vi "Set ADC.vi"(8 "error in (no error)":errorcluster, 9 "Data Rate":T1, 10 "Configure NAU7802":T2={"PGA"=enum."x1", "LDOVoltage"=enum."2.7"}, 11 "NAU7802 in":refnum<class "Adafruit NAU7802 24bit Strain Gauge.lvclass">) -> (0 "error out":errorcluster, 3 "NAU7802 out":refnum<class "Adafruit NAU7802 24bit Strain Gauge.lvclass">)   [LabVIEW 2020, in "CTI-Peripheral.lvlib" / "Adafruit NAU7802 24bit Strain Gauge.lvclass"]
uses:
  Adafruit NAU7802 24bit Strain Gauge.lvclass
  Private/ConfigData.ctl
  Private/NAU7802PGA.ctl
  Private/NAU7802LDOVoltage.ctl
  Private/NAU7802DataRate.ctl
  Adafruit NAU7802 24bit Strain Gauge.lvclass/Adafruit NAU7802 24bit Strain Gauge.ctl
  CTI/I2C Connection/I2C Connection.lvclass/I2C Connection.ctl
  CTI/Session/I2C Write Data.vi
  CTI/Session/I2C Read Data.vi
  CTI/I2C Connection/I2C Connection.lvclass
panel:
  out "Data":string
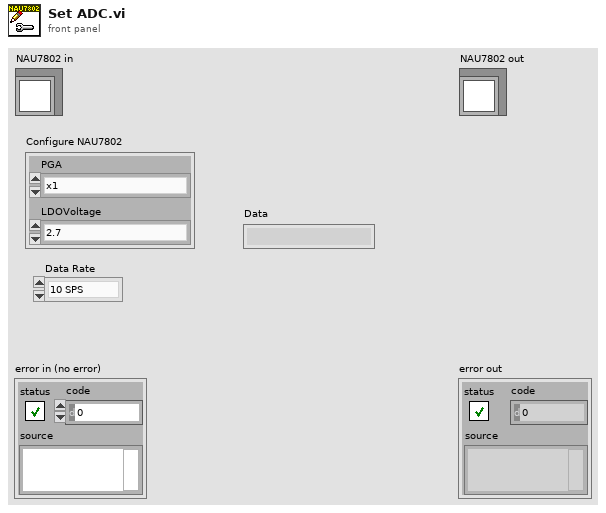
[diagram p1: front panel]
types:
  T1 = typedef "CTI-Peripheral.lvlib/Adafruit NAU7802 24bit Strain Gauge.lvclass/NAU7802DataRate.ctl" = enum16{"10 SPS", "20 SPS", "40 SPS", "80 SPS", "320 SPS"}
  T2 = typedef "ConfigData.ctl" = cluster{"PGA":T3, "LDOVoltage":T4}
  T3 = typedef "CTI-Peripheral.lvlib/Adafruit NAU7802 24bit Strain Gauge.lvclass/NAU7802PGA.ctl" = enum16{"x1", "x2", "x4", "x8", "x16", "x32", "x64", "x128"}
  T4 = typedef "CTI-Peripheral.lvlib/Adafruit NAU7802 24bit Strain Gauge.lvclass/NAU7802LDOVoltage.ctl" = enum16{"2.4", "2.7", "3.0", "3.3", "3.6", "3.9", "4.2", "4.5"}
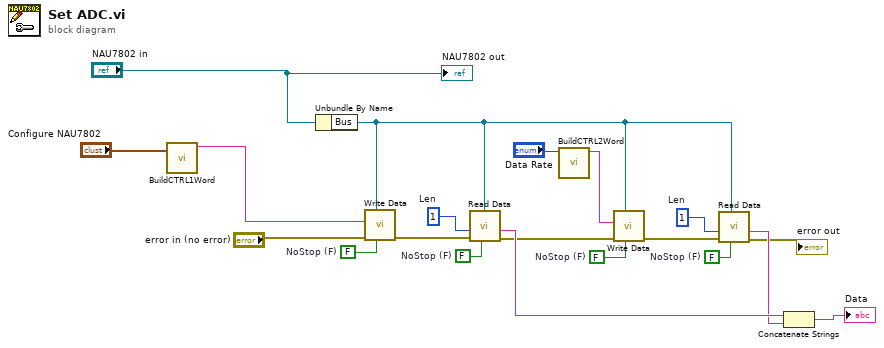
[diagram p0: block diagram]
diagram:
  w10 = FALSE  # NoStop (F)
  w9 = u8 1  # Len
  w8 = FALSE  # NoStop (F)
  w17 = FALSE  # NoStop (F)
  w18 = u8 1  # Len
  w19 = FALSE  # NoStop (F)
  n1 = call "BuildCTRL1Word.vi"("NewVal"="Configure NAU7802") -> ("string"=w15:string)  [unwired: 10 in]
  n2 = Unbundle By Name("NAU7802 in") -> ("Bus"=w6:refnum<class "I2C Connection.lvclass">)
  n3 = call "Write Data.vi"("NoStop (F)"=w19, "I2C Connection"=w6, "error in (no error)"="error in (no error)", "Data"=w15) -> ("error out"=w16:errorcluster)  [unwired: 7 in]
  n4 = call "Read Data.vi"("NoStop (F)"=w17, "I2C Connection"=w6, "error in (no error)"=w16, "Len"=w18) -> ("error out"=w7:errorcluster, "Data"=w14:string)  [unwired: 6 in]
  n5 = call "BuildCTRL2Word.vi"("NewVal"="Data Rate") -> ("string"=w4:string)  [unwired: 10 in]
  n6 = call "Write Data.vi"("NoStop (F)"=w8, "I2C Connection"=w6, "error in (no error)"=w7, "Data"=w4) -> ("error out"=w11:errorcluster)  [unwired: 7 in]
  n7 = call "Read Data.vi"("NoStop (F)"=w10, "I2C Connection"=w6, "error in (no error)"=w11, "Len"=w9) -> ("error out"=→"error out":errorcluster, "Data"=w2:string)  [unwired: 6 in]
  n8 = Concatenate Strings(w14, w2) -> (→"Data":string)
  "NAU7802 out" <- "NAU7802 in"
